vi "Check TE Controller Ports.vi"(7 "Refs":T1 {"Current Settings"."Pump" items=["Pump 0", "Pump 1", "Pump 2", "Pump 3", "Pump 4", "Pump 5"]; "Current Settings"."Chart X axis Timescale" min=20 max=180 step=1; "Current Settings"."RunTime Mode Settings"."Exp. Gas Tank" items=["0.07", "0.031", "0.877", "1.863", "3.881", "5.790", "7.688", "6.000"]; "Current Settings"."RunTime Mode Settings"."Insp. Gas Tank" items=["0.07", "0.031", "0.877", "1.863", "3.881", "5.790", "7.688", "6.000"]; "Current Settings"."RunTime Mode Settings"."I:E Ratio" max=30 scale=0.0..7.0; "Current Settings"."RunTime Mode Settings"."Resp Rate Brpm" min=0 max=30 format="%.2f"; "Current Settings"."TE#2 Configuration"."Serial Port"."XOFF Char" format="%.0x"; "Current Settings"."TE#2 Configuration"."Serial Port"."XON Char" format="%.0x"; "Current Settings"."TE#2 Configuration"."Serial Port"."flow control" items=["None"=0, "XON/XOFF"=1, "RTS/CTS"=2, "DTR/DSR"=4]; "Current Settings"."TE#2 Configuration"."Serial Port"."stop bits" items=["1.0"=10, "1.5"=15, "2.0"=20]; "Current Settings"."TE#2 Configuration"."Serial Port"."data bits" min=5 max=8 step=1; "Current Settings"."TE#2 Configuration"."Serial Port"."baud rate" items=["75"=75, "110"=110, "134"=134, "150"=150, "300"=300, "600"=600, "1200"=1200, "1800"=1800, "2400"=2400, "4800"=4800, "7200"=7200, "9600"=9600, "14400"=14400, "19200"=19200, "28800"=28800, "38400"=38400, "56000"=56000, "57600"=57600, "115200"=115200, "128000"=128000, "230400"=230400]; "Current Settings"."TE#2 Configuration"."Serial Port"."termination char" format="%.0x"; "Current Settings"."TE#1 Configuration"."Serial Port"."XOFF Char" format="%.0x"; "Current Settings"."TE#1 Configuration"."Serial Port"."XON Char" format="%.0x"; "Current Settings"."TE#1 Configuration"."Serial Port"."flow control" items=["None"=0, "XON/XOFF"=1, "RTS/CTS"=2, "DTR/DSR"=4]; "Current Settings"."TE#1 Configuration"."Serial Port"."stop bits" items=["1.0"=10, "1.5"=15, "2.0"=20]; "Current Settings"."TE#1 Configuration"."Serial Port"."data bits" min=5 max=8 step=1; "Current Settings"."TE#1 Configuration"."Serial Port"."baud rate" items=["75"=75, "110"=110, "134"=134, "150"=150, "300"=300, "600"=600, "1200"=1200, "1800"=1800, "2400"=2400, "4800"=4800, "7200"=7200, "9600"=9600, "14400"=14400, "19200"=19200, "28800"=28800, "38400"=38400, "56000"=56000, "57600"=57600, "115200"=115200, "128000"=128000, "230400"=230400]; "Current Settings"."TE#1 Configuration"."Serial Port"."termination char" format="%.0x"; "Current Settings"."Capnometer Configuration"."Device" items=["None", "TidalWave", "LoFlow / Canary", "Capnogard"]; "Current Settings"."Capnometer Configuration"."Serial Port"."XOFF Char" format="%.0x"; "Current Settings"."Capnometer Configuration"."Serial Port"."XON Char" format="%.0x"; "Current Settings"."Capnometer Configuration"."Serial Port"."flow control" items=["None"=0, "XON/XOFF"=1, "RTS/CTS"=2, "DTR/DSR"=4]; "Current Settings"."Capnometer Configuration"."Serial Port"."stop bits" items=["1.0"=10, "1.5"=15, "2.0"=20]; "Current Settings"."Capnometer Configuration"."Serial Port"."data bits" min=5 max=8 step=1; "Current Settings"."Capnometer Configuration"."Serial Port"."baud rate" items=["75"=75, "110"=110, "134"=134, "150"=150, "300"=300, "600"=600, "1200"=1200, "1800"=1800, "2400"=2400, "4800"=4800, "7200"=7200, "9600"=9600, "14400"=14400, "19200"=19200, "28800"=28800, "38400"=38400, "56000"=56000, "57600"=57600, "115200"=115200, "128000"=128000, "230400"=230400]; "Current Settings"."Capnometer Configuration"."Serial Port"."termination char" format="%.0x"; "Current Settings"."DAQx Settings"."Analog Output Settings (Volts)" format="%#.3g"; "Current Settings"."DAQx Settings"."Duty Cycle" min=10.0 max=90.0 format="%.1g"; "Current Settings"."DAQx Settings"."Frequency" min=20.0 max=200.0; "Current Settings"."DataLogging Settings"."Data File Duration (Minutes)" min=2 max=200 format="%#.2g"; "Current Settings"."Calibration Settings"."Tolerance #2" min=2 max=4096; "Current Settings"."Calibration Settings"."Cal. Average" min=2 max=4096; "Current Settings"."Test Settings"."Test Sensor ID" items=["(select)", "RB", "YC", "", "Other"]}, 9 "input cluster":T2={"Loaded Settings File"=path "", "Test Settings"={"Dual Channel"=FALSE, "Air Pump"=FALSE, "Optical Drive"=FALSE, "Pulsed Drive"=FALSE, "Calibration Mode"=FALSE, "Test Sensor ID"=0, "Test Chamber"="", "Test Operator"="", "Sample Descriptor"="", "Notes"=""}, "Calibration Settings"={"Cal. Average"=2, "Cal Averaging"=FALSE, "Tolerance #0"=0.0, "Tolerance #7"=0.0, "Tolerance #6"=0.0, "Tolerance #5"=0.0, "Tolerance #4"=0.0, "Tolerance #3"=0.0, "Tolerance #2"=0.0, "Tolerance #1"=0.0, "Gas Tank Settings"={"Gas Conc. #0"="", "Gas Conc. #1"=0.0, "Gas Conc. #2"=0.0, "Gas Conc. #3"=0.0, "Gas Conc. #4"=0.0, "Gas Conc. #5"=0.0, "Gas Conc. #6"=0.0, "Gas Conc. #7"=0.0}}, "DataLogging Settings"={"Data File Path"=path "c:/data", "Data File Duration (Minutes)"=2.0, "Log Filename"="Test Log.csv", "Config Path"=path ""}, "DAQx Settings"={"DAQ Device"="USBXDAQ", "Frequency"=20.0, "Duty Cycle"=50.0, "Analog Output Settings (Volts)"=[]}, "Capnometer Configuration"={"Serial Port"={"termination char"=10, "End read on termination character?"=TRUE, "Enabled?"=FALSE, "VISA resource name"="COM7", "baud rate"=9600, "data bits"=8, "parity"=enum."None", "stop bits"=10, "flow control"=0, "timeout (ms)"=10000, "Input buffer size"=4096, "End write on termination character?"=FALSE, "XON Char"=17, "XOFF Char"=19}, "Baro Pressure"=760, "Device"=0}, "TE#1 Configuration"={"Temp Set Point"=0.0, "Serial Port"={"termination char"=10, "End read on termination character?"=TRUE, "Enabled?"=FALSE, "VISA resource name"="COM1", "baud rate"=9600, "data bits"=8, "parity"=enum."None", "stop bits"=10, "flow control"=0, "timeout (ms)"=10000, "Input buffer size"=4096, "End write on termination character?"=TRUE, "XON Char"=17, "XOFF Char"=19}}, "TE#2 Configuration"={"Temp Set Point"=0.0, "Serial Port"={"termination char"=10, "End read on termination character?"=TRUE, "Enabled?"=FALSE, "VISA resource name"="COM1", "baud rate"=9600, "data bits"=8, "parity"=enum."None", "stop bits"=10, "flow control"=0, "timeout (ms)"=10000, "Input buffer size"=4096, "End write on termination character?"=TRUE, "XON Char"=17, "XOFF Char"=19}}, "RunTime Mode Settings "={"Resp Rate Brpm "=0.0, "I:E Ratio"=0, "Insp. Gas Tank"=0, "Exp. Gas Tank"=7}, "Chart X axis Timescale"=20, "Pump"=0} {"Pump" items=["Pump 0", "Pump 1", "Pump 2", "Pump 3", "Pump 4", "Pump 5"]; "Chart X axis Timescale" min=20 max=180 step=1; "RunTime Mode Settings"."Exp. Gas Tank" items=["0.07", "0.031", "0.877", "1.863", "3.881", "5.790", "7.688", "6.000"]; "RunTime Mode Settings"."Insp. Gas Tank" items=["0.07", "0.031", "0.877", "1.863", "3.881", "5.790", "7.688", "6.000"]; "RunTime Mode Settings"."I:E Ratio" max=30 scale=0.0..7.0; "RunTime Mode Settings"."Resp Rate Brpm" min=0 max=30 format="%.2f"; "TE#2 Configuration"."Serial Port"."XOFF Char" format="%.0x"; "TE#2 Configuration"."Serial Port"."XON Char" format="%.0x"; "TE#2 Configuration"."Serial Port"."flow control" items=["None"=0, "XON/XOFF"=1, "RTS/CTS"=2, "DTR/DSR"=4]; "TE#2 Configuration"."Serial Port"."stop bits" items=["1.0"=10, "1.5"=15, "2.0"=20]; "TE#2 Configuration"."Serial Port"."data bits" min=5 max=8 step=1; "TE#2 Configuration"."Serial Port"."baud rate" items=["75"=75, "110"=110, "134"=134, "150"=150, "300"=300, "600"=600, "1200"=1200, "1800"=1800, "2400"=2400, "4800"=4800, "7200"=7200, "9600"=9600, "14400"=14400, "19200"=19200, "28800"=28800, "38400"=38400, "56000"=56000, "57600"=57600, "115200"=115200, "128000"=128000, "230400"=230400]; "TE#2 Configuration"."Serial Port"."termination char" format="%.0x"; "TE#1 Configuration"."Serial Port"."XOFF Char" format="%.0x"; "TE#1 Configuration"."Serial Port"."XON Char" format="%.0x"; "TE#1 Configuration"."Serial Port"."flow control" items=["None"=0, "XON/XOFF"=1, "RTS/CTS"=2, "DTR/DSR"=4]; "TE#1 Configuration"."Serial Port"."stop bits" items=["1.0"=10, "1.5"=15, "2.0"=20]; "TE#1 Configuration"."Serial Port"."data bits" min=5 max=8 step=1; "TE#1 Configuration"."Serial Port"."baud rate" items=["75"=75, "110"=110, "134"=134, "150"=150, "300"=300, "600"=600, "1200"=1200, "1800"=1800, "2400"=2400, "4800"=4800, "7200"=7200, "9600"=9600, "14400"=14400, "19200"=19200, "28800"=28800, "38400"=38400, "56000"=56000, "57600"=57600, "115200"=115200, "128000"=128000, "230400"=230400]; "TE#1 Configuration"."Serial Port"."termination char" format="%.0x"; "Capnometer Configuration"."Device" items=["None", "TidalWave", "LoFlow / Canary", "Capnogard"]; "Capnometer Configuration"."Serial Port"."XOFF Char" format="%.0x"; "Capnometer Configuration"."Serial Port"."XON Char" format="%.0x"; "Capnometer Configuration"."Serial Port"."flow control" items=["None"=0, "XON/XOFF"=1, "RTS/CTS"=2, "DTR/DSR"=4]; "Capnometer Configuration"."Serial Port"."stop bits" items=["1.0"=10, "1.5"=15, "2.0"=20]; "Capnometer Configuration"."Serial Port"."data bits" min=5 max=8 step=1; "Capnometer Configuration"."Serial Port"."baud rate" items=["75"=75, "110"=110, "134"=134, "150"=150, "300"=300, "600"=600, "1200"=1200, "1800"=1800, "2400"=2400, "4800"=4800, "7200"=7200, "9600"=9600, "14400"=14400, "19200"=19200, "28800"=28800, "38400"=38400, "56000"=56000, "57600"=57600, "115200"=115200, "128000"=128000, "230400"=230400]; "Capnometer Configuration"."Serial Port"."termination char" format="%.0x"; "DAQx Settings"."Analog Output Settings (Volts)" format="%#.3g"; "DAQx Settings"."Duty Cycle" min=10.0 max=90.0 format="%.1g"; "DAQx Settings"."Frequency" min=20.0 max=200.0; "DataLogging Settings"."Data File Duration (Minutes)" min=2 max=200 format="%#.2g"; "Calibration Settings"."Tolerance #2" min=2 max=4096; "Calibration Settings"."Cal. Average" min=2 max=4096; "Test Settings"."Test Sensor ID" items=["(select)", "RB", "YC", "", "Other"]}, 10 "TE Controller 2 Configuration":T4={"termination char"=10, "End read on termination character?"=FALSE, "Enabled?"=TRUE, "VISA resource name"="COM4", "baud rate"=115200, "data bits"=8, "parity"=enum."None", "stop bits"=10, "flow control"=0, "timeout (ms)"=1, "Input buffer size"=4096, "End write on termination character?"=FALSE, "XON Char"=17, "XOFF Char"=19} {"XOFF Char" format="%.0x"; "XON Char" format="%.0x"; "flow control" items=["None"=0, "XON/XOFF"=1, "RTS/CTS"=2, "DTR/DSR"=4]; "stop bits" items=["1.0"=10, "1.5"=15, "2.0"=20]; "data bits" min=5 max=8 step=1; "baud rate" items=["75"=75, "110"=110, "134"=134, "150"=150, "300"=300, "600"=600, "1200"=1200, "1800"=1800, "2400"=2400, "4800"=4800, "7200"=7200, "9600"=9600, "14400"=14400, "19200"=19200, "28800"=28800, "38400"=38400, "56000"=56000, "57600"=57600, "115200"=115200, "128000"=128000, "230400"=230400]; "termination char" format="%.0x"}, 11 "TE Controller 1 Configuration":T4={"termination char"=10, "End read on termination character?"=FALSE, "Enabled?"=TRUE, "VISA resource name"="COM3", "baud rate"=115200, "data bits"=8, "parity"=enum."None", "stop bits"=10, "flow control"=0, "timeout (ms)"=1, "Input buffer size"=4096, "End write on termination character?"=FALSE, "XON Char"=17, "XOFF Char"=19} {"XOFF Char" format="%.0x"; "XON Char" format="%.0x"; "flow control" items=["None"=0, "XON/XOFF"=1, "RTS/CTS"=2, "DTR/DSR"=4]; "stop bits" items=["1.0"=10, "1.5"=15, "2.0"=20]; "data bits" min=5 max=8 step=1; "baud rate" items=["75"=75, "110"=110, "134"=134, "150"=150, "300"=300, "600"=600, "1200"=1200, "1800"=1800, "2400"=2400, "4800"=4800, "7200"=7200, "9600"=9600, "14400"=14400, "19200"=19200, "28800"=28800, "38400"=38400, "56000"=56000, "57600"=57600, "115200"=115200, "128000"=128000, "230400"=230400]; "termination char" format="%.0x"}) -> (3 "input cluster 2":T2={"Loaded Settings File"=path "", "Test Settings"={"Dual Channel"=FALSE, "Air Pump"=FALSE, "Optical Drive"=FALSE, "Pulsed Drive"=FALSE, "Calibration Mode"=FALSE, "Test Sensor ID"=0, "Test Chamber"="", "Test Operator"="", "Sample Descriptor"="", "Notes"=""}, "Calibration Settings"={"Cal. Average"=2, "Cal Averaging"=FALSE, "Tolerance #0"=0.0, "Tolerance #7"=0.0, "Tolerance #6"=0.0, "Tolerance #5"=0.0, "Tolerance #4"=0.0, "Tolerance #3"=0.0, "Tolerance #2"=0.0, "Tolerance #1"=0.0, "Gas Tank Settings"={"Gas Conc. #0"="", "Gas Conc. #1"=0.0, "Gas Conc. #2"=0.0, "Gas Conc. #3"=0.0, "Gas Conc. #4"=0.0, "Gas Conc. #5"=0.0, "Gas Conc. #6"=0.0, "Gas Conc. #7"=0.0}}, "DataLogging Settings"={"Data File Path"=path "c:/data", "Data File Duration (Minutes)"=2.0, "Log Filename"="Test Log.csv", "Config Path"=path ""}, "DAQx Settings"={"DAQ Device"="USBXDAQ", "Frequency"=20.0, "Duty Cycle"=50.0, "Analog Output Settings (Volts)"=[]}, "Capnometer Configuration"={"Serial Port"={"termination char"=10, "End read on termination character?"=TRUE, "Enabled?"=FALSE, "VISA resource name"="COM7", "baud rate"=9600, "data bits"=8, "parity"=enum."None", "stop bits"=10, "flow control"=0, "timeout (ms)"=10000, "Input buffer size"=4096, "End write on termination character?"=FALSE, "XON Char"=17, "XOFF Char"=19}, "Baro Pressure"=760, "Device"=0}, "TE#1 Configuration"={"Temp Set Point"=0.0, "Serial Port"={"termination char"=10, "End read on termination character?"=TRUE, "Enabled?"=FALSE, "VISA resource name"="COM1", "baud rate"=9600, "data bits"=8, "parity"=enum."None", "stop bits"=10, "flow control"=0, "timeout (ms)"=10000, "Input buffer size"=4096, "End write on termination character?"=TRUE, "XON Char"=17, "XOFF Char"=19}}, "TE#2 Configuration"={"Temp Set Point"=0.0, "Serial Port"={"termination char"=10, "End read on termination character?"=TRUE, "Enabled?"=FALSE, "VISA resource name"="COM1", "baud rate"=9600, "data bits"=8, "parity"=enum."None", "stop bits"=10, "flow control"=0, "timeout (ms)"=10000, "Input buffer size"=4096, "End write on termination character?"=TRUE, "XON Char"=17, "XOFF Char"=19}}, "RunTime Mode Settings "={"Resp Rate Brpm "=0.0, "I:E Ratio"=0, "Insp. Gas Tank"=0, "Exp. Gas Tank"=7}, "Chart X axis Timescale"=20, "Pump"=0} {"Pump" items=["Pump 0", "Pump 1", "Pump 2", "Pump 3", "Pump 4", "Pump 5"]; "Chart X axis Timescale" min=20 max=180 step=1; "RunTime Mode Settings"."Exp. Gas Tank" items=["0.07", "0.031", "0.877", "1.863", "3.881", "5.790", "7.688", "6.000"]; "RunTime Mode Settings"."Insp. Gas Tank" items=["0.07", "0.031", "0.877", "1.863", "3.881", "5.790", "7.688", "6.000"]; "RunTime Mode Settings"."I:E Ratio" max=30 scale=0.0..7.0; "RunTime Mode Settings"."Resp Rate Brpm" min=0 max=30 format="%.2f"; "TE#2 Configuration"."Serial Port"."XOFF Char" format="%.0x"; "TE#2 Configuration"."Serial Port"."XON Char" format="%.0x"; "TE#2 Configuration"."Serial Port"."flow control" items=["None"=0, "XON/XOFF"=1, "RTS/CTS"=2, "DTR/DSR"=4]; "TE#2 Configuration"."Serial Port"."stop bits" items=["1.0"=10, "1.5"=15, "2.0"=20]; "TE#2 Configuration"."Serial Port"."data bits" min=5 max=8 step=1; "TE#2 Configuration"."Serial Port"."baud rate" items=["75"=75, "110"=110, "134"=134, "150"=150, "300"=300, "600"=600, "1200"=1200, "1800"=1800, "2400"=2400, "4800"=4800, "7200"=7200, "9600"=9600, "14400"=14400, "19200"=19200, "28800"=28800, "38400"=38400, "56000"=56000, "57600"=57600, "115200"=115200, "128000"=128000, "230400"=230400]; "TE#2 Configuration"."Serial Port"."termination char" format="%.0x"; "TE#1 Configuration"."Serial Port"."XOFF Char" format="%.0x"; "TE#1 Configuration"."Serial Port"."XON Char" format="%.0x"; "TE#1 Configuration"."Serial Port"."flow control" items=["None"=0, "XON/XOFF"=1, "RTS/CTS"=2, "DTR/DSR"=4]; "TE#1 Configuration"."Serial Port"."stop bits" items=["1.0"=10, "1.5"=15, "2.0"=20]; "TE#1 Configuration"."Serial Port"."data bits" min=5 max=8 step=1; "TE#1 Configuration"."Serial Port"."baud rate" items=["75"=75, "110"=110, "134"=134, "150"=150, "300"=300, "600"=600, "1200"=1200, "1800"=1800, "2400"=2400, "4800"=4800, "7200"=7200, "9600"=9600, "14400"=14400, "19200"=19200, "28800"=28800, "38400"=38400, "56000"=56000, "57600"=57600, "115200"=115200, "128000"=128000, "230400"=230400]; "TE#1 Configuration"."Serial Port"."termination char" format="%.0x"; "Capnometer Configuration"."Device" items=["None", "TidalWave", "LoFlow / Canary", "Capnogard"]; "Capnometer Configuration"."Serial Port"."XOFF Char" format="%.0x"; "Capnometer Configuration"."Serial Port"."XON Char" format="%.0x"; "Capnometer Configuration"."Serial Port"."flow control" items=["None"=0, "XON/XOFF"=1, "RTS/CTS"=2, "DTR/DSR"=4]; "Capnometer Configuration"."Serial Port"."stop bits" items=["1.0"=10, "1.5"=15, "2.0"=20]; "Capnometer Configuration"."Serial Port"."data bits" min=5 max=8 step=1; "Capnometer Configuration"."Serial Port"."baud rate" items=["75"=75, "110"=110, "134"=134, "150"=150, "300"=300, "600"=600, "1200"=1200, "1800"=1800, "2400"=2400, "4800"=4800, "7200"=7200, "9600"=9600, "14400"=14400, "19200"=19200, "28800"=28800, "38400"=38400, "56000"=56000, "57600"=57600, "115200"=115200, "128000"=128000, "230400"=230400]; "Capnometer Configuration"."Serial Port"."termination char" format="%.0x"; "DAQx Settings"."Analog Output Settings (Volts)" format="%#.3g"; "DAQx Settings"."Duty Cycle" min=10.0 max=90.0 format="%.1g"; "DAQx Settings"."Frequency" min=20.0 max=200.0; "DataLogging Settings"."Data File Duration (Minutes)" min=2 max=200 format="%#.2g"; "Calibration Settings"."Tolerance #2" min=2 max=4096; "Calibration Settings"."Cal. Average" min=2 max=4096; "Test Settings"."Test Sensor ID" items=["(select)", "RB", "YC", "", "Other"]})   [LabVIEW 2016]
uses:
  Controls/Serial Visa Control.ctl
  Controls/UI Settings.ctl
  Controls/Aux CO2 Control.ctl
  Controls/Aux CO2 Selector.ctl
  Controls/Aux TE Control.ctl
  Controls/DAQ Needed.ctl
  Controls/Processed Variables.ctl
  Controls/AirPump Controls.ctl
  Controls/IE Ratio knob.ctl
  Controls/Queues And Others.ctl
  Controls/SerialPortControl.ctl
panel:
  in  "Tab Control":enum32{"Stopped", "Running"}(tab)
  in  "Run Button":bool
  in  "OK Button":bool
  in  "Stop Button 2":bool
  out "T1 Temperature":sgl[][](graph)
  out "ReadData":sgl[][](array[numeric]) format="%.2g"
  in  "SetPoint#2":sgl format="%.2g"
  out "bytes read":i16
  in  "Custom Text":string
  in  "Command":u16(ring) items=["<Select>", "$R0=", "$R101?", "$R102?", "$R105?", "Custom User Entry"]
  out "Array":bool[](array[boolean])
  out "Data Received":i16[](graph)
  in  "SetPoint#1":sgl format="%.2g"
  in  "Retrieve Button":bool
  in  "Send Button":bool
  in  "Stop Button":bool
  in  "Start Button":bool
  in  "Count":dbl
  out "TE Controller Latest Data":string[](array[string])
  out "TE Controller Returned Data Log":string[](array[string])
  # "Note: Setting Brpm to zero will\ndisable Insp / Exp digital output."
  # "mmHg"
  # "pts"
  # "tolerance"
  # "AN5 (Temp 1)"
  # "AN6 (Temp 2)"
  # "AN7 (Temp 3)"
  # "AN8 (T FET)"
  # "AN0 (T POT)"
  # "Tref (Set Pt))"
  # "(Spare)"
  # "Note: Setting Brpm to zero will\ndisable Insp / Exp digital output."
  # "mmHg"
  # "pts"
  # "tolerance"
  # "Note: Setting Brpm to zero will\ndisable Insp / Exp digital output."
  # "mmHg"
  # "pts"
  # "tolerance"
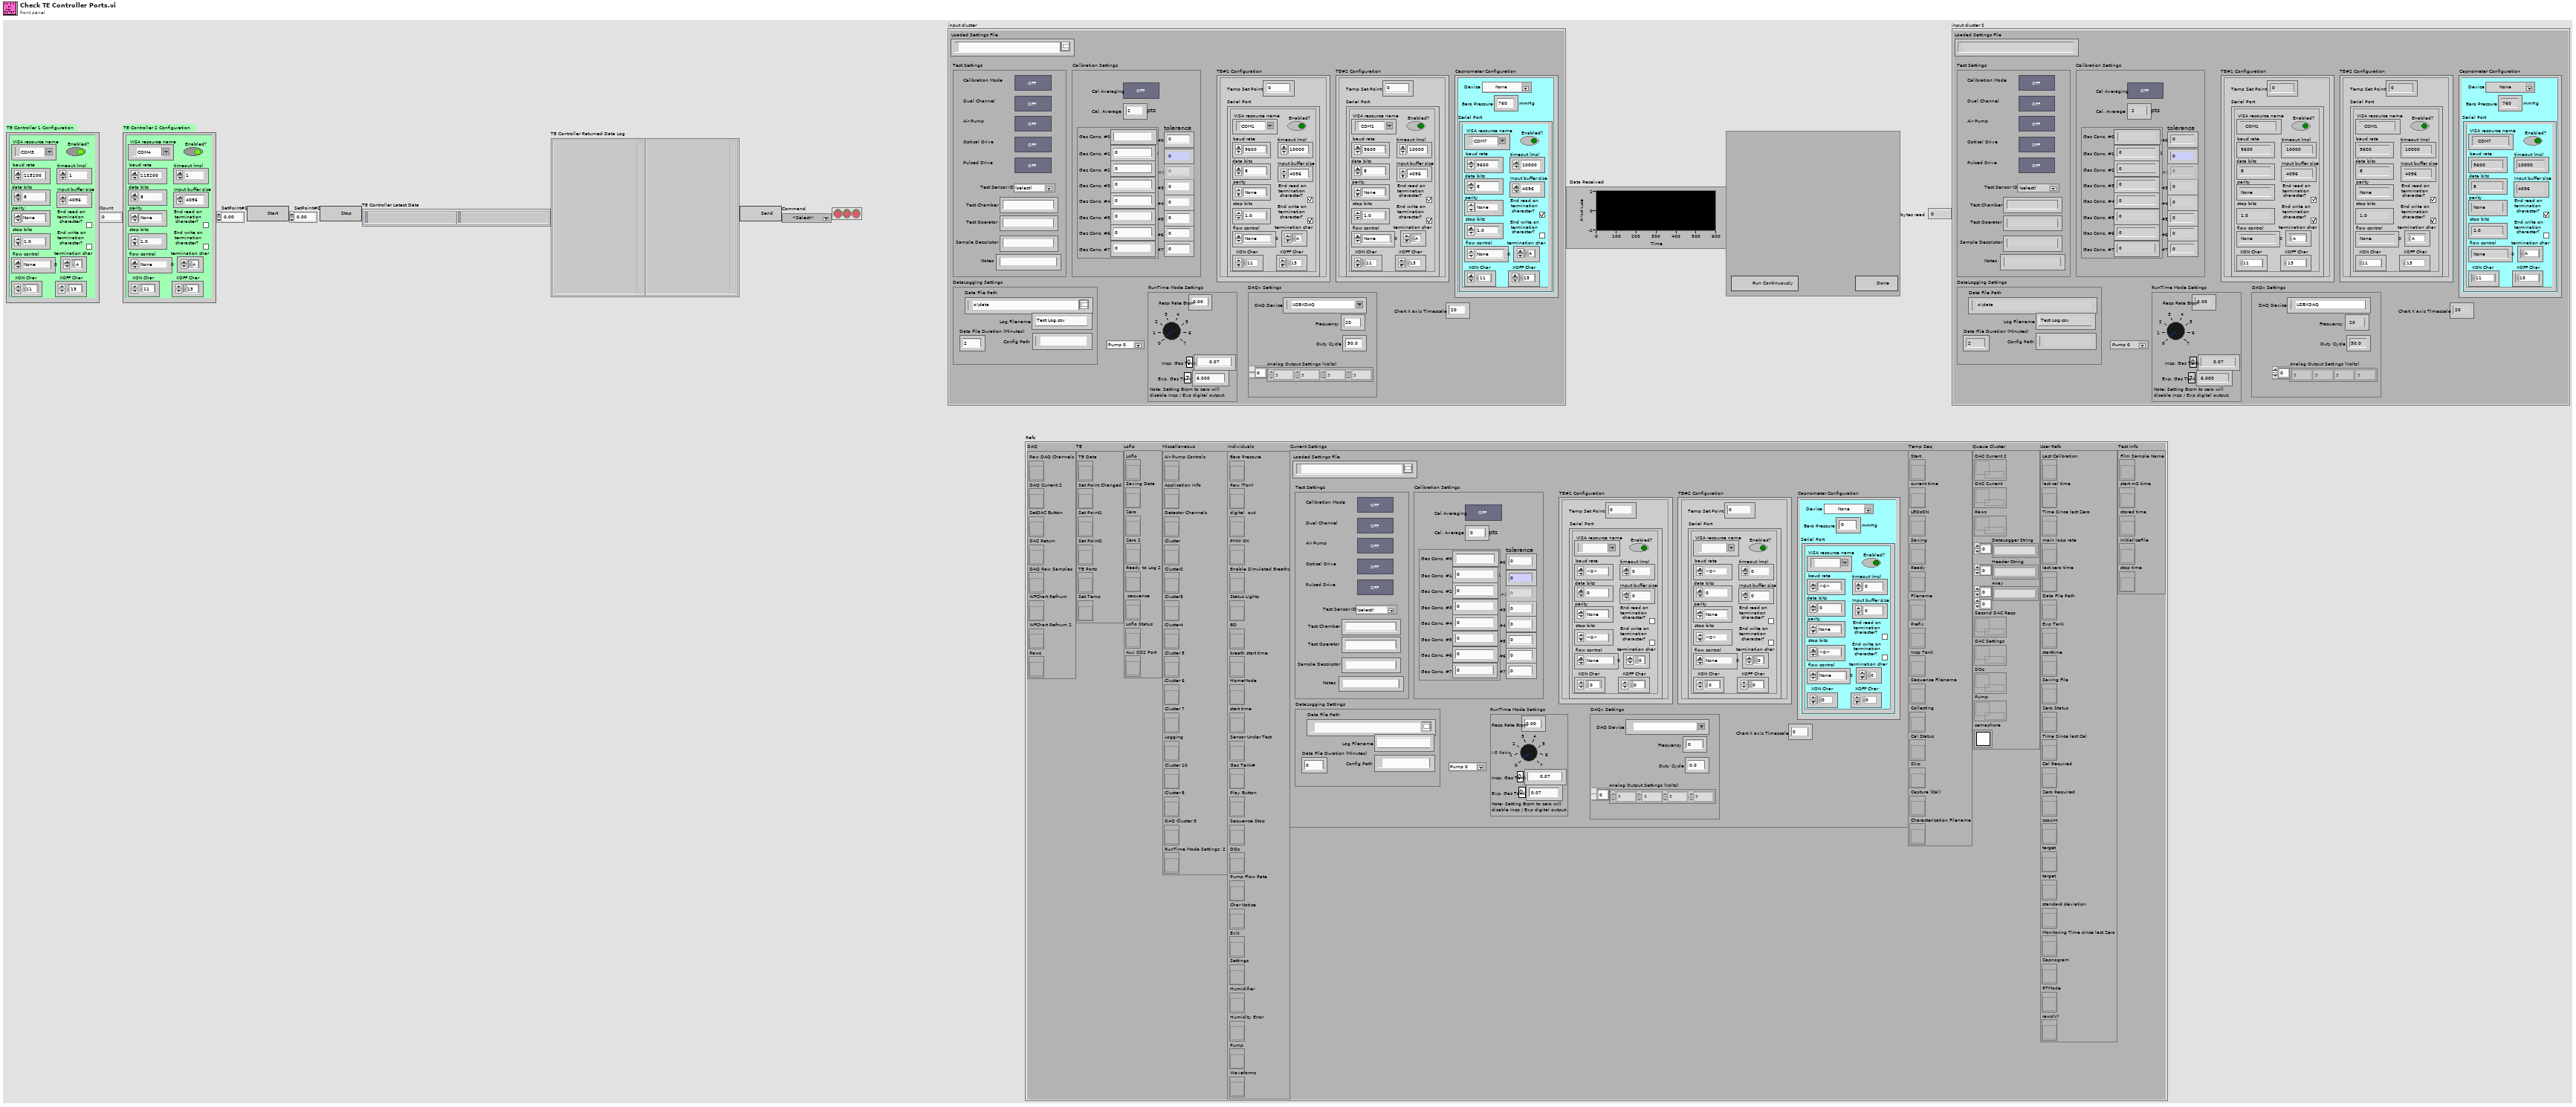
[diagram p1: front panel]
types:
  T1 = typedef "DAQ Needed.ctl" = cluster{"DAQ":cluster{"Raw DAQ Channels":refnum<vi>, "DAQ Current 2":refnum<vi>, "SetDAC Button":refnum<vi>, "DAC Return":refnum<vi>, "DAQ Raw Samples":refnum<vi>, "WFChart Refnum":refnum<vi>, "WFChart Refnum 2":refnum<vi>, "Raws":refnum<vi>}, "TE":cluster{"TE Data":refnum<vi>, "Set Point Changed":refnum<vi>, "Set Point1":refnum<vi>, "Set Point2":refnum<vi>, "TE Ports":refnum<vi>, "Set Temp":refnum<vi>}, "Loflo":cluster{"Loflo":refnum<vi>, "Saving Data":refnum<vi>, "Zero":refnum<vi>, "Zero 2":refnum<vi>, "Ready to Log 2":refnum<vi>, " sequence":refnum<vi>, "Loflo Status ":refnum<vi>, "Aux CO2 Port":refnum<vi>}, "Miscellaneous":cluster{"Air Pump Controls":refnum<vi>, "Application Info":refnum<vi>, "Detector Channels ":refnum<vi>, "Cluster":refnum<vi>, "Cluster2":refnum<vi>, "Cluster3":refnum<vi>, "Cluster4":refnum<vi>, "Cluster 5":refnum<vi>, "Cluster 6":refnum<vi>, "Cluster 7":refnum<vi>, "Logging":refnum<vi>, "Cluster 10":refnum<vi>, "Cluster 8":refnum<vi>, "DAQ Cluster 3":refnum<vi>, "RunTime Mode Settings  2":refnum<vi>}, "Individuals":cluster{"Baro Pressure":refnum<vi>, "Raw (Torr)":refnum<vi>, "digital  out":refnum<vi>, "PMW OK":refnum<vi>, "Enable Simulated Breaths":refnum<vi>, "Status Lights":refnum<vi>, "BD":refnum<vi>, "breath start time":refnum<vi>, "HomeMode":refnum<vi>, "start time":refnum<vi>, "Sensor Under Test":refnum<vi>, "Gas Tank#":refnum<vi>, "Play Button":refnum<vi>, "Sequence Stop":refnum<vi>, "DOs":refnum<vi>, "Pump Flow Rate":refnum<vi>, "Char Notice":refnum<vi>, "Exit":refnum<vi>, "Settings":refnum<vi>, "Humidifier":refnum<vi>, "Humidity Error":refnum<vi>, "Pump":refnum<vi>, "Waveforms":refnum<vi>}, "Current Settings":T2, "Temp Seq":cluster{"Start":refnum<vi>, "current time":refnum<vi>, "LEDsON":refnum<vi>, "Saving":refnum<vi>, "Ready":refnum<vi>, "Filename":refnum<vi>, "Prefix":refnum<vi>, "Insp Tank":refnum<vi>, "Sequence Filename":refnum<vi>, "Collecting":refnum<vi>, "Cal Status":refnum<vi>, "Skip":refnum<vi>, "Capture (Cal)":refnum<vi>, "Characterization Filename":refnum<vi>}, "Queue Cluster":T7, "User Refs":cluster{"Last Calibration":refnum<vi>, "last cal time":refnum<vi>, "Time Since last Zero":refnum<vi>, "main loop rate":refnum<vi>, "last zero time":refnum<vi>, "Data File Path":refnum<vi>, "Exp Tank":refnum<vi>, "starttime":refnum<vi>, "Saving File":refnum<vi>, "Zero Status":refnum<vi>, "Time Since last Cal":refnum<vi>, "Cal Required":refnum<vi>, "Zero Required":refnum<vi>, "zcount":refnum<vi>, "target":refnum<vi>, "target":refnum<vi>, "standard deviation":refnum<vi>, "Monitoring Time since last Zero":refnum<vi>, "Capnogram":refnum<vi>, "RTMode":refnum<vi>, "raws(V)":refnum<vi>}, "Test Info":cluster{"Film Sample Name":refnum<vi>, "start mS time":refnum<vi>, "stored time":refnum<vi>, "InitializeFile":refnum<vi>, "stop time":refnum<vi>}}
  T2 = typedef "UI Settings.ctl" = cluster{"Loaded Settings File":path, "Test Settings":cluster{"Dual Channel":bool, "Air Pump":bool, "Optical Drive":bool, "Pulsed Drive":bool, "Calibration Mode":bool, "Test Sensor ID":u16, "Test Chamber":string, "Test Operator":string, "Sample Descriptor":string, "Notes":string}, "Calibration Settings":cluster{"Cal. Average":u16, "Cal Averaging":bool, "Tolerance #0":sgl, "Tolerance #7":sgl, "Tolerance #6":sgl, "Tolerance #5":sgl, "Tolerance #4":sgl, "Tolerance #3":sgl, "Tolerance #2":sgl, "Tolerance #1":sgl, "Gas Tank Settings":cluster{"Gas Conc. #0":string, "Gas Conc. #1":sgl, "Gas Conc. #2":sgl, "Gas Conc. #3":sgl, "Gas Conc. #4":sgl, "Gas Conc. #5":sgl, "Gas Conc. #6":sgl, "Gas Conc. #7":sgl}}, "DataLogging Settings":cluster{"Data File Path":path, "Data File Duration (Minutes)":sgl, "Log Filename":string, "Config Path":path}, "DAQx Settings":cluster{"DAQ Device":tag, "Frequency":dbl, "Duty Cycle":dbl, "Analog Output Settings (Volts)":sgl[]}, "Capnometer Configuration":T3, "TE#1 Configuration":T6, "TE#2 Configuration":T6, "RunTime Mode Settings ":cluster{"Resp Rate Brpm ":sgl, "I:E Ratio":u8, "Insp. Gas Tank":u16, "Exp. Gas Tank":u16}, "Chart X axis Timescale":u16, "Pump":u16}
  T3 = typedef "Aux CO2 Control.ctl" = cluster{"Serial Port":T4, "Baro Pressure":u32, "Device":T5}
  T4 = typedef "Serial Visa Control.ctl" = cluster{"termination char":u8, "End read on termination character?":bool, "Enabled?":bool, "VISA resource name":refnum<visa-resource-name>, "baud rate":u32, "data bits":u16, "parity":enum16{"None", "Odd", "Even", "Mark", "Space"}, "stop bits":u16, "flow control":u16, "timeout (ms)":u32, "Input buffer size":u32, "End write on termination character?":bool, "XON Char":u8, "XOFF Char":u8}
  T5 = typedef "Aux CO2 Selector.ctl" = u16
  T6 = typedef "Aux TE Control.ctl" = cluster{"Temp Set Point":sgl, "Serial Port":T4}
  T7 = typedef "Queues And Others.ctl" = cluster{"DAC Current 2":refnum<queue>, "DAC Current":refnum<queue>, "Raws":refnum<queue>, "DataLogger String":string[], "Header String":string[], "Array":string[][], "Second DAC Resp":refnum<queue>, "DAC Settings":refnum<queue>, "DOs":refnum<queue>, "Pump":refnum<queue>, "semaphore":T8}
  T8 = typedef "Semaphore RefNum" = refnum<k1>
  T9 = typedef "SerialPortControl.ctl" = enum16{"Initialize", "Write Data", "Read Data", "Close Port"}
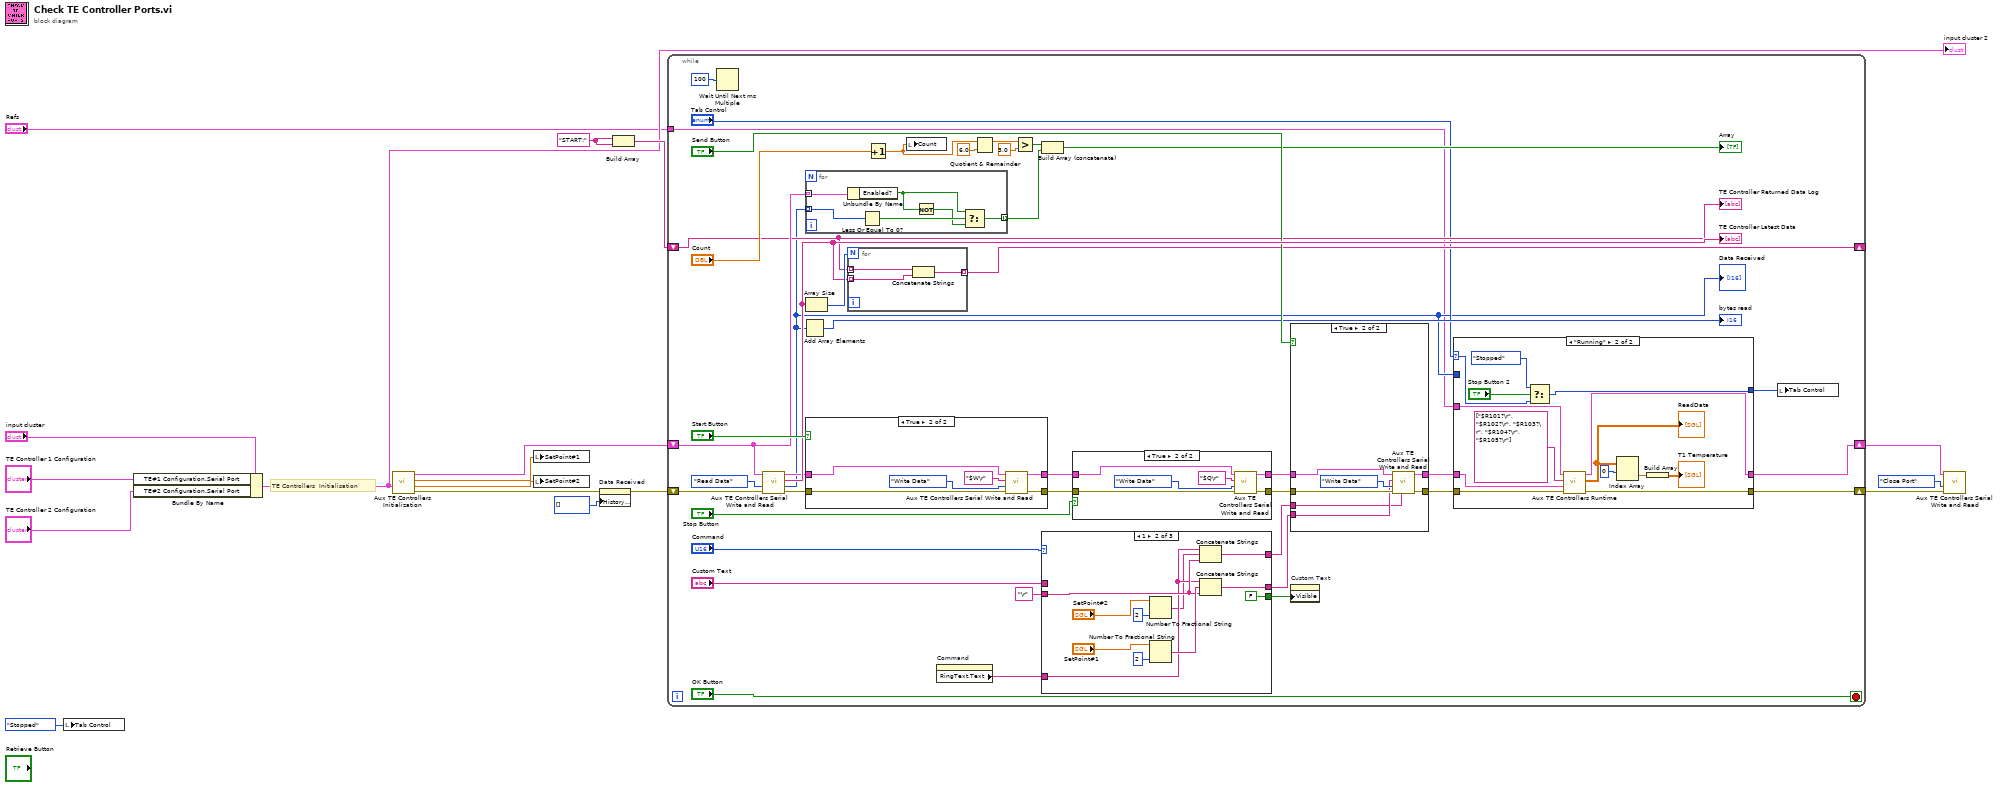
[diagram p0: block diagram]
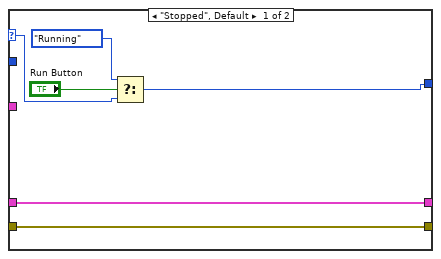
[diagram p2: hidden frame]
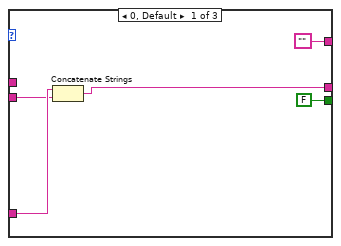
[diagram p3: hidden frame]
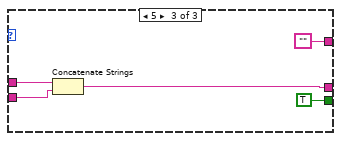
[diagram p4: hidden frame]
diagram:
  w13 = "START:"
  # "TE Controllers  Initialisation"
  n1 = local write "Tab Control"(enum32{"Stopped", "Running"}."Stopped" ("Tab Control")) -> ()
  n2 = Bundle By Name(cluster="input cluster", "TE#1 Configuration.Serial Port"="TE Controller 1 Configuration", "TE#2 Configuration.Serial Port"="TE Controller 2 Configuration") -> (w2:T2)
  "input cluster 2" <- w2
  n3 = call "Aux TE Controllers Initialization.vi"("input cluster"=w2) -> ("Error Out"=w9:errorcluster, "Temp Set Point 2"=w8:sgl, "Temp Set Point 1"=w7:sgl, "TE Serial Ports Out"=w10:T4[])  [unwired: 7 in]
  n4 = local write "SetPoint#1"(w7) -> ()
  n5 = local write "SetPoint#2"(w8) -> ()
  n6 = property on="Data Received" class="WFChart (strict)"(error in=w9, "History Data"=i16[] []) -> (error out=w11:errorcluster)  [unwired: 1 in, 1 out]
  n7 = Build Array(w13, w13) -> (w12:string[])
  n8 = while {
    shift-right: [w24] -> w15
    shift-left: w10 -> [w36]
    shift-right: [w23] -> w14
    shift-left: w11 -> [w56]
    shift-right: [w44] -> _
    shift-left: w12 -> [w29]
    tunnel: "Refs" -> [w18]
    stop <- "OK Button" stop-if-true
    n9 = Wait Until Next ms Multiple(millisecond multiple=100) -> ()  [unwired: 1 out]
    n10 = call "Aux TE Controllers Serial Write and Read.vi"("error in"=w56, "Action"=SerialPortControl."Read Data", "TE Controller Serial Ports In"=w36) -> ("Error Out"=w54:errorcluster, "#Bytes R/W"=w20:i16[], "Data Read"=w53:string[], "TE Controller Serial Ports Out"=w52:T4[])  [unwired: 2 in, 1 out]
    "TE Controller Latest Data" <- w53
    "Data Received" <- w20
    n11 = Add Array Elements(numeric array=w20) -> (sum=→"bytes read":i16)
    n12 = for {
      tunnel: w36 -> [w106] mode=indexing
      tunnel: [w102] -> w35 mode=indexing
      tunnel: w20 -> [w105] mode=indexing
      n13 = Unbundle By Name(w106) -> ("Enabled?"=w103:bool)
      n14 = Less Or Equal To 0?(x=w105) -> (x <= 0?=w104:bool)
      n15 = Not(x=w103) -> (.not. x?=w101:bool)
      n16 = Select(t=w103, s=w104, f=w101) -> (s? t:f=w102:bool)
    }
    n17 = Array Size(array=w53) -> (size(s)=w59:i32)
    n18 = case shown="True" "Start Button" {
      tunnel: [w125 w129] -> w51
      tunnel: w54 -> [w125 w128]
      tunnel: [w124 w126] -> w50
      tunnel: w52 -> [w124 w127]
      frame False {
      }
      frame True {
        n19 = call "Aux TE Controllers Serial Write and Read.vi"("error in"=w128, "Action"=SerialPortControl."Write Data", "string to write"="$W\r", "TE Controller Serial Ports In"=w127) -> ("Error Out"=w129:errorcluster, "TE Controller Serial Ports Out"=w126:T4[])  [unwired: 1 in, 3 out]
      }
    }
    n20 = for {
      N: w59 -> [_]
      tunnel: w53 -> [w133] mode=indexing
      tunnel: w29 -> [w132] mode=indexing
      tunnel: [w134] -> w44 mode=indexing
      n21 = Concatenate Strings(w132, w133) -> (w134:string)
    }
    n22 = Increment(x="Count") -> (x+1=w42:dbl)
    n23 = local write "Count"(w42) -> ()
    n24 = property on="Command" class="Ring (strict)"() -> ("RingText.Text"=w33:string)  [unwired: 2 in, 2 out]
    n25 = Quotient & Remainder(x=w42, y=6.0) -> (x-y*floor(x/y)=w40:dbl)  [unwired: 1 out]
    n26 = Greater?(x=w40, y=3.0) -> (0:w38:bool)
    n27 = Build Array (concatenate)(w38, w35) -> (→"Array":bool[])
    n28 = case shown="1" "Command" {
      tunnel: [w84 w95 w100] -> w27
      tunnel: w33 -> [w83 w86 _]
      tunnel: "\r" ("string to write") -> [w82 w88 w98]
      tunnel: "Custom Text" -> [_ _ w99]
      tunnel: [FALSE FALSE TRUE] -> w30
      tunnel: ["" w87 ""] -> w19
      frame 0, Default {
        n29 = Concatenate Strings(w83, w82) -> (w84:string)
      }
      frame 1 {
        n30 = Number To Fractional String(number="SetPoint#2", precision (6)=i16 2) -> (F-format string=w85:string)  [unwired: 2 in]
        n31 = Number To Fractional String(number="SetPoint#1", precision (6)=i16 2) -> (F-format string=w93:string)  [unwired: 2 in]
        n32 = Concatenate Strings(w86, w85, w88) -> (w87:string)
        n33 = Concatenate Strings(w86, w93, w88) -> (w95:string)
      }
      frame 5 {
        n34 = Concatenate Strings(w99, w98) -> (w100:string)
      }
    }
    n35 = case shown="True" "Stop Button" {
      tunnel: [w117 w121] -> w47
      tunnel: w51 -> [w117 w120]
      tunnel: [w116 w118] -> w48
      tunnel: w50 -> [w116 w119]
      frame False {
      }
      frame True {
        n36 = call "Aux TE Controllers Serial Write and Read.vi"("error in"=w120, "Action"=SerialPortControl."Write Data", "string to write"="$Q\r", "TE Controller Serial Ports In"=w119) -> ("Error Out"=w121:errorcluster, "TE Controller Serial Ports Out"=w118:T4[])  [unwired: 1 in, 3 out]
      }
    }
    n37 = case shown="True" "Send Button" {
      tunnel: [w108 w114] -> w21
      tunnel: w47 -> [w108 w113]
      tunnel: [w107 w111] -> w22
      tunnel: w48 -> [w107 w112]
      tunnel: w27 -> [_ w110]
      tunnel: w19 -> [_ w109]
      frame False {
      }
      frame True {
        n38 = call "Aux TE Controllers Serial Write and Read.vi"("second string"=w109, "error in"=w113, "Action"=SerialPortControl."Write Data", "string to write"=w110, "TE Controller Serial Ports In"=w112) -> ("Error Out"=w114:errorcluster, "TE Controller Serial Ports Out"=w111:T4[])  [unwired: 3 out]
      }
    }
    n39 = property on="Custom Text" class="Str"("Visible"=w30) -> ()  [unwired: 2 in, 2 out]
    n40 = case shown="\"Running\"" "Tab Control" {
      selector: "Tab Control" -> [w64 w78]
      tunnel: [w65 w76] -> w25
      tunnel: w22 -> [w60 w75]
      tunnel: w21 -> [w61 w74]
      tunnel: [w61 w71] -> w23
      tunnel: [w60 w72] -> w24
      tunnel: w20 -> [_ _]
      tunnel: w18 -> [_ w66]
      frame "Stopped", Default {
        n41 = Select(t=enum32{"Stopped", "Running"}."Running" ("Tab Control"), s="Run Button", f=w64) -> (s? t:f=w65:enum32{"Stopped", "Running"})
      }
      frame "Running" {
        n42 = Select(t=enum32{"Stopped", "Running"}."Stopped" ("Tab Control"), s="Stop Button 2", f=w78) -> (s? t:f=w76:enum32{"Stopped", "Running"})
        n43 = call "Aux TE Controllers Runtime.vi"("Error In"=w74, "TE Serial Ports In"=w75, "CmdsToWrite"=string[] ["$R101?\r", "$R102?\r", "$R103?\r", "$R104?\r", "$R105?\r"], "Refs"=w66) -> ("Error Out"=w71:errorcluster, "ReadData"=w69:sgl[][], "TE Serial Ports Out"=w72:T4[])  [unwired: 5 out]
        "ReadData" <- w69
        n44 = Index Array(array=w69, index (row)=0) -> (element=w70:sgl[])  [unwired: 1 in]
        n45 = Build Array(w70) -> (→"T1 Temperature":sgl[][])
      }
    }
    n46 = local write "Tab Control"(w25) -> ()
    "TE Controller Returned Data Log" <- w29
  }
  n47 = call "Aux TE Controllers Serial Write and Read.vi"("error in"=w14, "Action"=SerialPortControl."Close Port", "TE Controller Serial Ports In"=w15) -> ()  [unwired: 2 in, 5 out]
